vi "Fail If Error.vi"(7 "Description":string, 8 "error in (no error)":errorcluster, 10 "Assert error":errorcluster, 11 "LUnit Test Case In":refnum<class "LUnit Test Case V2.lvclass">) -> (0 "error out":errorcluster, 3 "LUnit Test Case Out":refnum<class "LUnit Test Case V2.lvclass">)   [LabVIEW 2020, in "LUnit Test Case V2.lvclass"]
doc: "Generates a fail result for the calling test method if the inputs contains an error with status \"True\". A description may be provided to the result."
uses:
  LUnit Test Case V2.lvclass
  LUnit Test Case V2.lvclass/LUnit Test Case V2.ctl
  Private/Append Result.vi
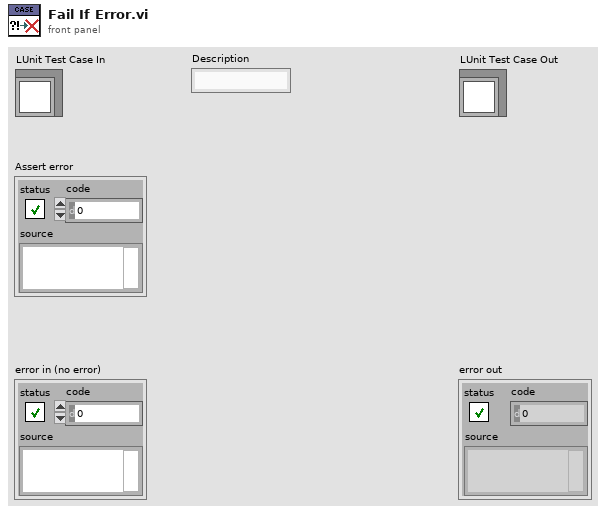
[diagram p1: front panel]
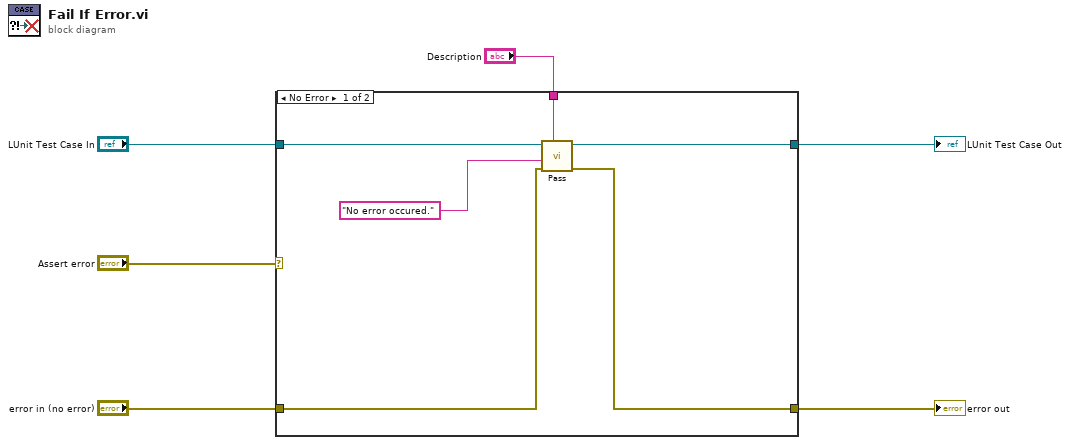
[diagram p0: block diagram]
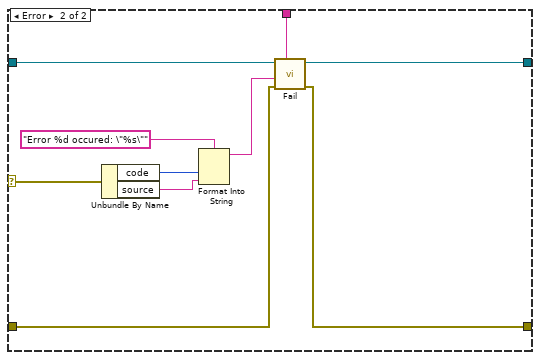
[diagram p2: hidden frame]
diagram:
  n1 = case shown="No Error" "Assert error" {
    selector: "Assert error" -> [_ w19]
    tunnel: "LUnit Test Case In" -> [w12 w22]
    tunnel: [w11 w21] -> w4
    tunnel: [w10 w20] -> w3
    tunnel: "Description" -> [w9 w16]
    tunnel: "error in (no error)" -> [w7 w13]
    frame No Error {
      n2 = call "Pass.vi"("Description"=w9, "error in (no error)"=w7, "Message"="No error occured.", "LUnit Test Case In"=w12) -> ("error out"=w10:errorcluster, "LUnit Test Case Out"=w11:refnum<class "LUnit Test Case V2.lvclass">)  [unwired: 6 in]
    }
    frame Error {
      n3 = Unbundle By Name(w19) -> ("code"=w15:i32, "source"=w14:string)
      n4 = Format Into String(format string="Error %d occured: \"%s\"", w15, w14) -> (resulting string=w18:string)  [unwired: 2 in, 1 out]
      n5 = call "Fail.vi"("Description"=w16, "error in (no error)"=w13, "Message"=w18, "LUnit Test Case In"=w22) -> ("error out"=w20:errorcluster, "LUnit Test Case Out"=w21:refnum<class "LUnit Test Case V2.lvclass">)  [unwired: 6 in]
    }
  }
  "error out" <- w3
  "LUnit Test Case Out" <- w4
